vi "Delete First Element.vi"(2 "Input Array":i32[](array[numeric])) -> (0 "Updated Array":i32[](array[numeric]))   [LabVIEW 2016]
doc: "This function deletes the first element of the input array"
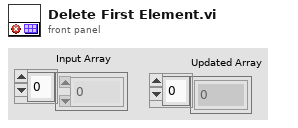
[diagram p1: front panel]
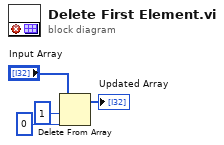
[diagram p0: block diagram]
diagram:
  n1 = Delete From Array(array="Input Array", length=1, index=0) -> (array with subset deleted=→"Updated Array":i32[])  [unwired: 1 out]
